vi "System Control Labview Programme.vi"() -> ()   [LabVIEW 2022 SP3]
uses:
  <vilib>/DAQmx/read.llb/DAQmx Read (Digital Bool 1Line 1Point).vi
  <vilib>/DAQmx/read.llb/DAQmx Read (Analog 1D DBL NChan 1Samp).vi
  <vilib>/DAQmx/create/channels.llb/DAQmx Create Channel (AI-Voltage-Basic).vi
  <vilib>/DAQmx/create/channels.llb/DAQmx Create Channel (DI-Digital Input).vi
  <vilib>/DAQmx/miscellaneous.llb/DAQmx Fill In Error Info.vi
panel:
  in  "Intensity":dbl
  out "Lux Meter":dbl
  out "Piezo Signal":dbl(graph)
  out "Train":bool
  out "Light On":bool
  out "Lux Metwer":dbl(knob) scale=0.0..700.0
  out "data":dbl[](array[numeric]) format="%0.2f"
  in  "Digital Input":tag
  out "Train detection":dbl
  out "IR":dbl
  in  "Numeric 3":dbl
  out "Connect":bool=TRUE
  in  "Numeric 2":dbl
  out "Power On":bool=TRUE
  in  "Numeric Main":dbl
  in  "VISA resource":refnum<visa-resource-name>
  in  "Connect":bool
  in  "Power on":bool
  # "STREET LIGHTING SYSTEM"
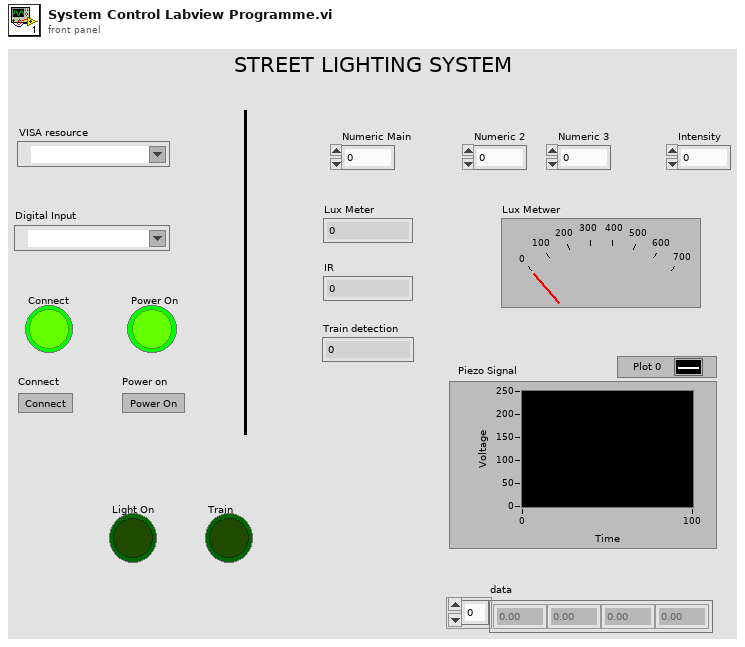
[diagram p1: front panel]
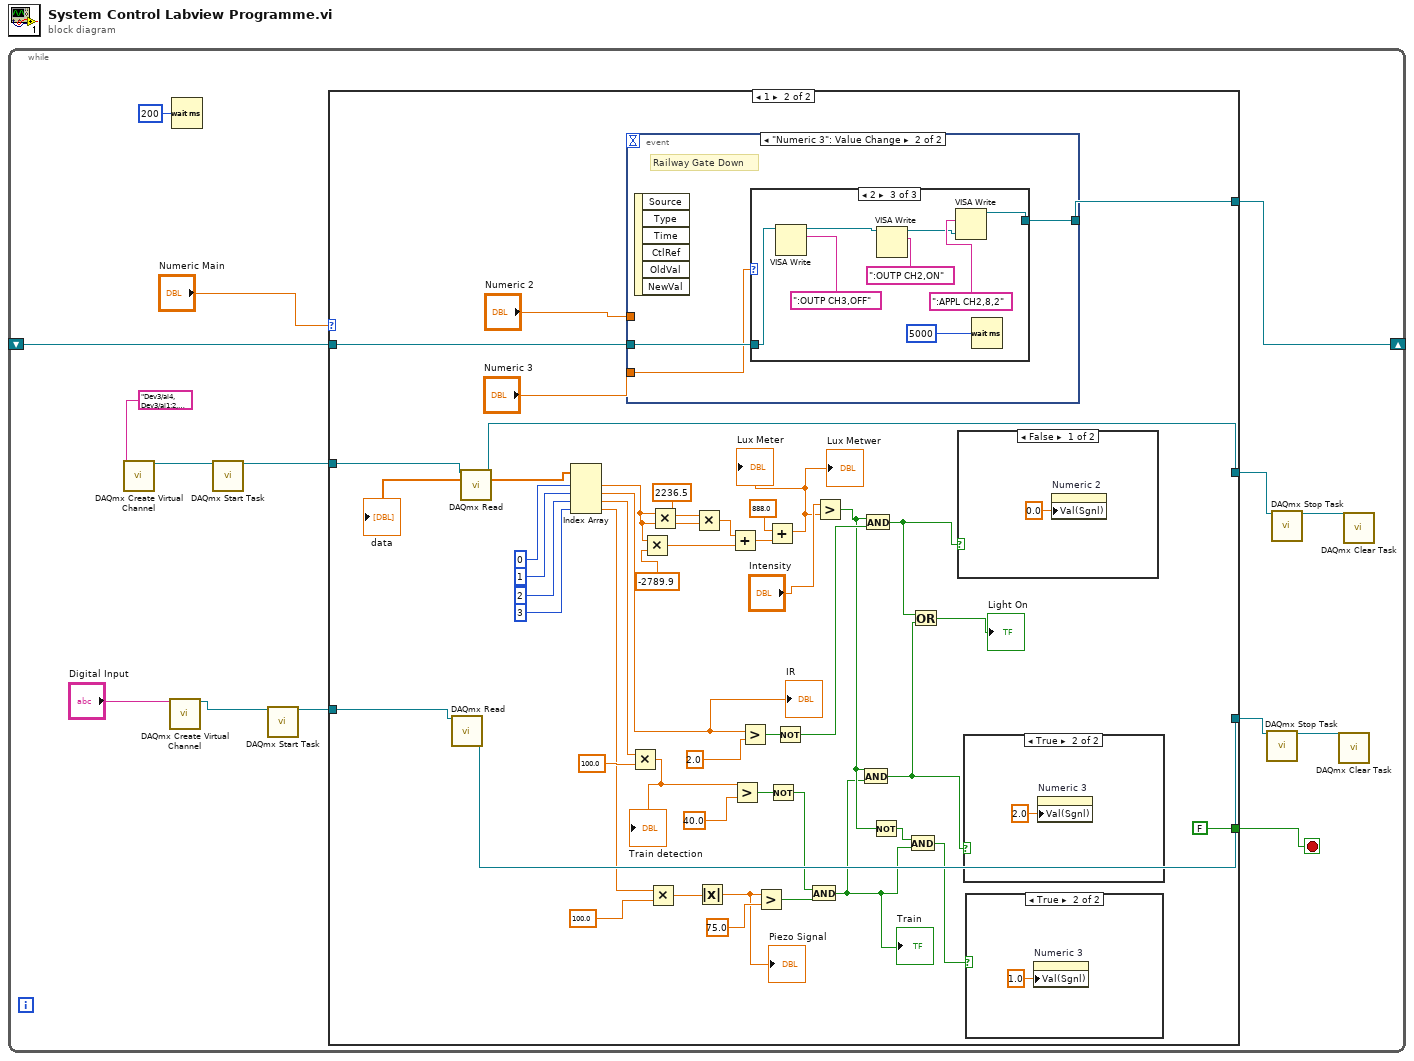
[diagram p0: block diagram]
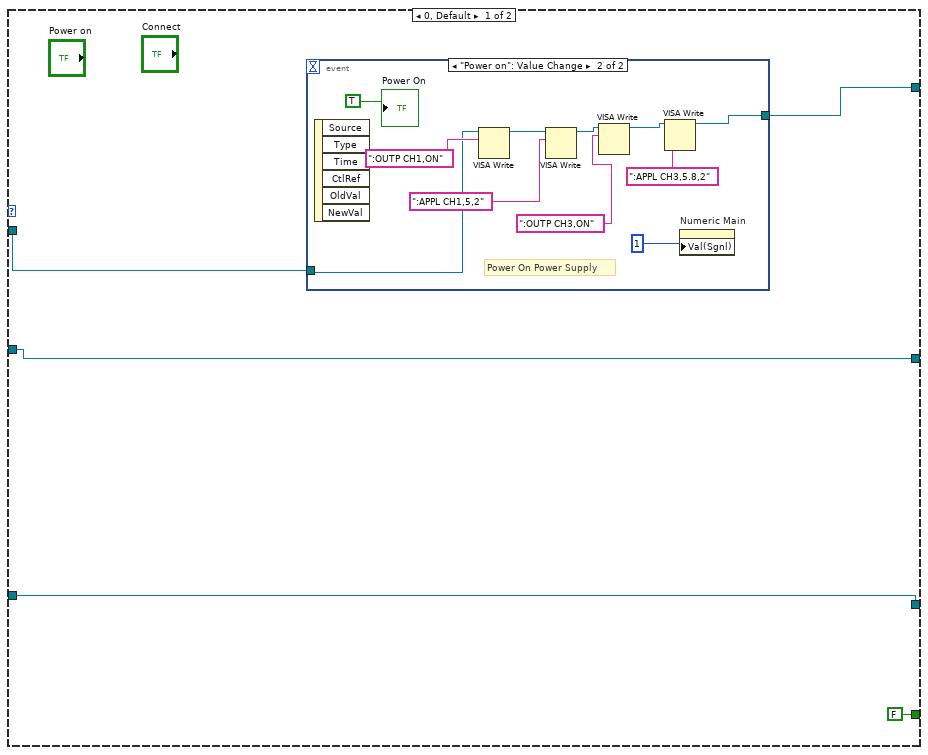
[diagram p2: hidden frame]
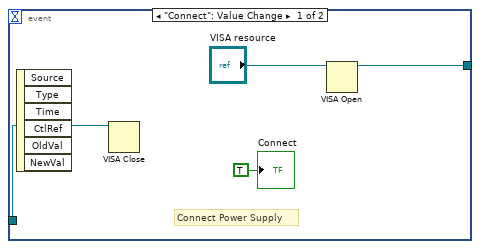
[diagram p3: hidden frame]
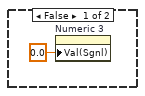
[diagram p5: hidden frame]
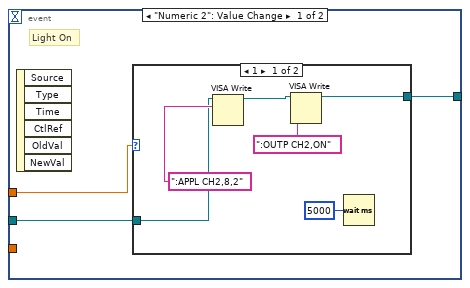
[diagram p6: hidden frame]
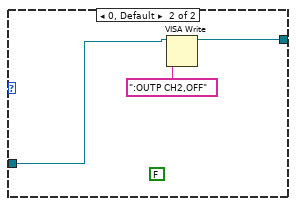
[diagram p7: hidden frame]
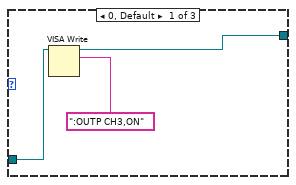
[diagram p8: hidden frame]
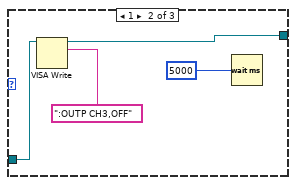
[diagram p9: hidden frame]
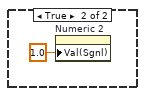
[diagram p10: hidden frame]
diagram:
  n1 = while {
    shift-right: [w13] -> _
    shift-left: _ -> [w14]
    stop <- w9 stop-if-true
    n2 = call-poly <vilib>:"DAQmx Create Virtual Channel.vi"("physical channels"=tag "Dev3/ai4, Dev3/ai1:2, Dev3/ai7") -> ("task out"=w12:refnum<k21>)  [unwired: 13 in, 1 out]
    n3 = call-poly <vilib>:"DAQmx Create Virtual Channel.vi"("lines"="Digital Input") -> ("task out"=w5:refnum<k21>)  [unwired: 13 in, 1 out]
    n4 = Wait (ms)(milliseconds to wait=u32 200) -> ()  [unwired: 1 out]
    n5 = call <vilib>:"DAQmx Start Task.vi"("task/channels in"=w12) -> ("task out"=w11:refnum<k21>)  [unwired: 13 in, 1 out]
    n6 = call <vilib>:"DAQmx Start Task.vi"("task/channels in"=w5) -> ("task out"=w3:refnum<k21>)  [unwired: 13 in, 1 out]
    n7 = case shown="1" "Numeric Main" {
      tunnel: w14 -> [w20 w71]
      tunnel: [w19 w76] -> w13
      tunnel: w11 -> [w17 w82]
      tunnel: [FALSE FALSE] -> w9
      tunnel: [w17 w74] -> w8
      tunnel: w3 -> [w16 w69]
      tunnel: [w16 w68] -> w1
      frame 0, Default {
        n8 = event shown="[1] \"Power on\": Value Change" {
          selector: _ -> [_ _]
          dyn-events: _ -> [_ _]
          timeout: _ -> [_ _]
          tunnel: w20 -> [w23 w28]
          tunnel: [w22 w27] -> w19
          event "Connect": Value Change {
            # "Connect Power Supply"
            n9 = event-data() -> ()  [unwired: 1 in, 6 out]
            n10 = VISA Close(VISA resource name=w23) -> ()  [unwired: 1 in, 1 out]
            n11 = VISA Open(VISA resource name="VISA resource") -> (VISA resource name=w22:refnum<visa-resource-name>)  [unwired: 4 in, 1 out]
            "Connect" <- TRUE
          }
          event "Power on": Value Change {
            # "Power On Power Supply"
            n12 = event-data() -> ()  [unwired: 1 in, 6 out]
            n13 = VISA Write(VISA resource name=w28, write buffer=":OUTP CH1,ON") -> (VISA resource name out=w35:refnum<visa-resource-name>)  [unwired: 1 in, 2 out]
            n14 = VISA Write(VISA resource name=w35, write buffer=":APPL CH1,5,2") -> (VISA resource name out=w33:refnum<visa-resource-name>)  [unwired: 1 in, 2 out]
            n15 = VISA Write(VISA resource name=w33, write buffer=":OUTP CH3,ON") -> (VISA resource name out=w31:refnum<visa-resource-name>)  [unwired: 1 in, 2 out]
            n16 = VISA Write(VISA resource name=w31, write buffer=":APPL CH3,5.8,2") -> (VISA resource name out=w27:refnum<visa-resource-name>)  [unwired: 1 in, 2 out]
            n17 = property on="Numeric Main" class="DigNum (strict)"("Val(Sgnl)"=1) -> ()  [unwired: 2 in, 2 out]
            "Power On" <- TRUE
          }
        }
      }
      frame 1 {
        n18 = call-poly <vilib>:"DAQmx Read.vi"("task/channels in"=w69) -> ("task out"=w68:refnum<k21>)  [unwired: 12 in, 2 out]
        n19 = call-poly <vilib>:"DAQmx Read.vi"("task/channels in"=w82) -> ("task out"=w74:refnum<k21>, "data"=w81:dbl[])  [unwired: 12 in, 1 out]
        "data" <- w81
        n20 = Index Array(array=w81, index #1=0 ("index"), index #2=1 ("index"), index #3=2 ("index"), index #4=3 ("index")) -> (element #1=w45:dbl, element #2=w79:dbl, element #3=w67:dbl, element #4=w61:dbl)
        "IR" <- w79
        n21 = event shown="[1] \"Numeric 3\": Value Change" {
          selector: _ -> [_ _]
          dyn-events: _ -> [_ _]
          timeout: _ -> [_ _]
          tunnel: "Numeric 2" -> [w88 _]
          tunnel: w71 -> [w87 w100]
          tunnel: [w86 w99] -> w76
          tunnel: "Numeric 3" -> [_ w98]
          event "Numeric 2": Value Change {
            # "Light On"
            n22 = event-data() -> ()  [unwired: 1 in, 6 out]
            n23 = case shown="1" w88 {
              tunnel: w87 -> [w91 w95]
              tunnel: [w90 w96] -> w86
              frame 1 {
                n24 = VISA Write(VISA resource name=w91, write buffer=":APPL CH2,8,2") -> (VISA resource name out=w94:refnum<visa-resource-name>)  [unwired: 1 in, 2 out]
                n25 = VISA Write(VISA resource name=w94, write buffer=":OUTP CH2,ON") -> (VISA resource name out=w90:refnum<visa-resource-name>)  [unwired: 1 in, 2 out]
                n26 = Wait (ms)(milliseconds to wait=u32 5000) -> ()  [unwired: 1 out]
              }
              frame 0, Default {
                (unwired) FALSE
                n27 = VISA Write(VISA resource name=w95, write buffer=":OUTP CH2,OFF") -> (VISA resource name out=w96:refnum<visa-resource-name>)  [unwired: 1 in, 2 out]
              }
            }
          }
          event "Numeric 3": Value Change {
            # "Railway Gate Down"
            n28 = event-data() -> ()  [unwired: 1 in, 6 out]
            n29 = case shown="2" w98 {
              tunnel: w100 -> [w102 w105 w113]
              tunnel: [w101 w106 w108] -> w99
              frame 0, Default {
                n30 = VISA Write(VISA resource name=w102, write buffer=":OUTP CH3,ON") -> (VISA resource name out=w101:refnum<visa-resource-name>)  [unwired: 1 in, 2 out]
              }
              frame 1 {
                n31 = VISA Write(VISA resource name=w105, write buffer=":OUTP CH3,OFF") -> (VISA resource name out=w106:refnum<visa-resource-name>)  [unwired: 1 in, 2 out]
                n32 = Wait (ms)(milliseconds to wait=u32 5000) -> ()  [unwired: 1 out]
              }
              frame 2 {
                n33 = VISA Write(VISA resource name=w113, write buffer=":OUTP CH3,OFF") -> (VISA resource name out=w111:refnum<visa-resource-name>)  [unwired: 1 in, 2 out]
                n34 = VISA Write(VISA resource name=w111, write buffer=":OUTP CH2,ON") -> (VISA resource name out=w109:refnum<visa-resource-name>)  [unwired: 1 in, 2 out]
                n35 = VISA Write(VISA resource name=w109, write buffer=":APPL CH2,8,2") -> (VISA resource name out=w108:refnum<visa-resource-name>)  [unwired: 1 in, 2 out]
                n36 = Wait (ms)(milliseconds to wait=u32 5000) -> ()  [unwired: 1 out]
              }
            }
          }
        }
        n37 = Multiply(x=w67, y=100.0) -> (x*y=w66:dbl)
        "Train detection" <- w66
        n38 = Multiply(x=w45, y=-2789.9) -> (x*y=w44:dbl)
        n39 = Multiply(x=w61, y=100.0) -> (x*y=w59:dbl)
        n40 = Multiply(x=w45, y=w45) -> (x*y=w49:dbl)
        n41 = Multiply(x=w49, y=2236.5) -> (x*y=w43:dbl)
        n42 = Absolute Value(x=w59) -> (abs(x)=w55:dbl)
        "Piezo Signal" <- w55
        n43 = Add(x=w43, y=w44) -> (x+y=w42:dbl)
        n44 = Greater?(x=w66, y=40.0) -> (0:w72:bool)
        n45 = Greater?(x=w79, y=2.0) -> (0:w77:bool)
        n46 = Greater?(x=w55, y=75.0) -> (0:w57:bool)
        n47 = Add(x=w42, y=888.0) -> (x+y=w40:dbl)
        "Lux Metwer" <- w40
        "Lux Meter" <- w40
        n48 = Not(x=w72) -> (.not. x?=w56:bool)
        n49 = Not(x=w77) -> (.not. x?=w54:bool)
        n50 = And(x=w56, y=w57) -> (x .and. y?=w39:bool)
        "Train" <- w39
        n51 = Greater?(x="Intensity", y=w40) -> (0:w46:bool)
        n52 = And(x=w46, y=w39) -> (x .and. y?=w37:bool)
        n53 = And(x=w46, y=w54) -> (x .and. y?=w38:bool)
        n54 = Not(x=w46) -> (.not. x?=w53:bool)
        n55 = And(x=w53, y=w39) -> (x .and. y?=w52:bool)
        n56 = Or(x=w38, y=w37) -> (x .or. y?=→"Light On":bool)
        n57 = case shown="False" w38 {
          frame False {
            n58 = property on="Numeric 2" class="DigNum (strict)"("Val(Sgnl)"=0.0 ("Value (Signaling)")) -> ()  [unwired: 2 in, 2 out]
          }
          frame True {
            n59 = property on="Numeric 2" class="DigNum (strict)"("Val(Sgnl)"=1.0 ("Value (Signaling)")) -> ()  [unwired: 2 in, 2 out]
          }
        }
        n60 = case shown="True" w37 {
          frame False {
          }
          frame True {
            n61 = property on="Numeric 3" class="DigNum (strict)"("Val(Sgnl)"=2.0 ("Value (Signaling)")) -> ()  [unwired: 2 in, 2 out]
          }
        }
        n62 = case shown="True" w52 {
          frame False {
            n63 = property on="Numeric 3" class="DigNum (strict)"("Val(Sgnl)"=0.0 ("Value (Signaling)")) -> ()  [unwired: 2 in, 2 out]
          }
          frame True {
            n64 = property on="Numeric 3" class="DigNum (strict)"("Val(Sgnl)"=1.0 ("Value (Signaling)")) -> ()  [unwired: 2 in, 2 out]
          }
        }
      }
    }
    n65 = call <vilib>:"DAQmx Stop Task.vi"("task/channels in"=w1) -> ("task out"=w2:refnum<k21>)  [unwired: 13 in, 1 out]
    n66 = call <vilib>:"DAQmx Stop Task.vi"("task/channels in"=w8) -> ("task out"=w7:refnum<k21>)  [unwired: 13 in, 1 out]
    n67 = call <vilib>:"DAQmx Clear Task.vi"("task in"=w2) -> ()  [unwired: 14 in, 1 out]
    n68 = call <vilib>:"DAQmx Clear Task.vi"("task in"=w7) -> ()  [unwired: 14 in, 1 out]
  }
